vi "PolyGen.vi"() -> ()   [LabVIEW 2016]
uses:
  <vilib>/Utility/file.llb/Read Delimited Spreadsheet (string).vi
  <vilib>/Analysis/NI_AALPro.lvlib
panel:
  out "Z":cluster{dbl, dbl[]}[](array[cluster])
  out "X":cluster{dbl, dbl[]}[](array[cluster])
  out "Y":cluster{dbl, dbl[]}[](array[cluster])
  out "Application:Command Line Arguments":string[](array[string])
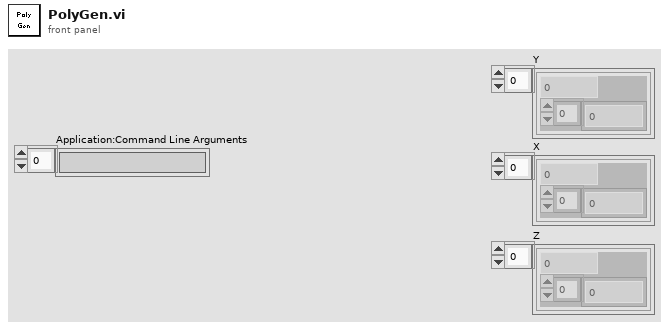
[diagram p1: front panel]
types:
  T1 = enum16{"open", "replace", "create", "open or create", "replace or create", "replace or create with confirmation"}
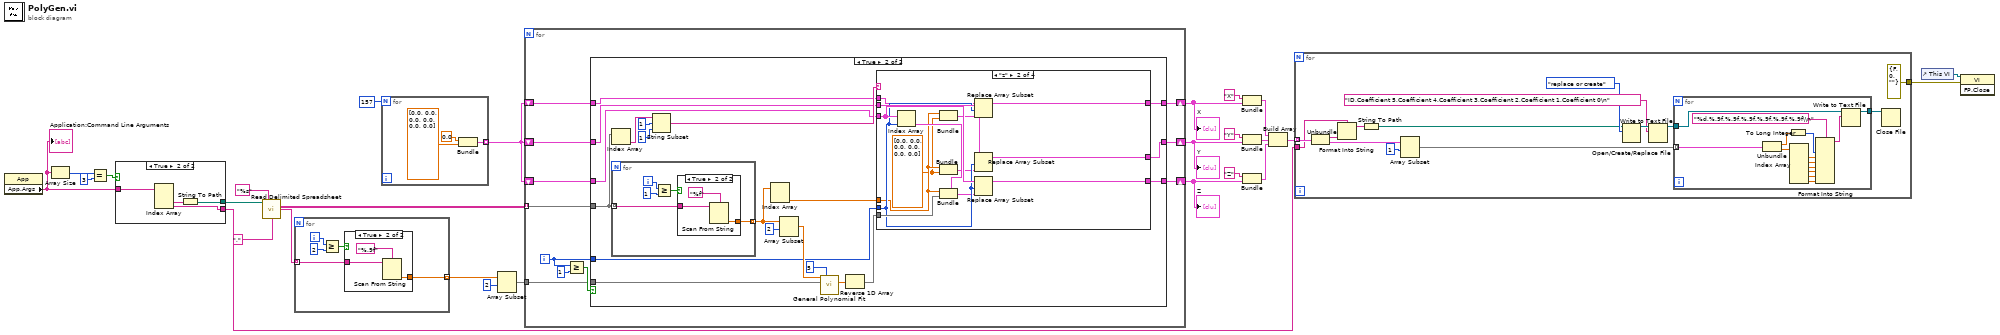
[diagram p0: block diagram]
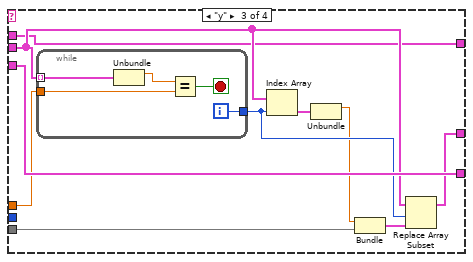
[diagram p4: hidden frame]
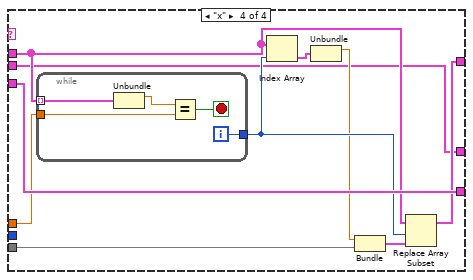
[diagram p5: hidden frame]
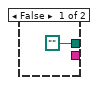
[diagram p8: hidden frame]
diagram:
  n1 = property class="App"() -> ("App.Args"=w24:string[])  [unwired: 2 in, 2 out]
  "Application:Command Line Arguments" <- w24
  n2 = Array Size(array=w24) -> (size(s)=w23:i32)
  n3 = Equal?(x=w23, y=3) -> (x = y?=w21:bool)
  n4 = case shown="True" w21 {
    tunnel: w24 -> [_ w32]
    tunnel: [path "" w31] -> w25
    tunnel: [_ w29] -> w3
    frame False {
    }
    frame True {
      n5 = Index Array(array=w32) -> (element #2=w30:string, element #3=w29:string)  [unwired: 3 in, 1 out]
      n6 = String To Path(string=w30) -> (path=w31:path)
    }
  }
  n7 = call-poly <vilib>:"Read Delimited Spreadsheet.vi"("file path (dialog if empty)"=w25, "format (%s)"="%s", "delimiter (\\t)"="," ("delimiter (\\t)")) -> ("all rows"=w17:string[][], "first row"=w20:string[])  [unwired: 7 in, 4 out]
  n8 = for {
    tunnel: w20 -> [w34] mode=indexing
    tunnel: [w33] -> w19 mode=indexing
    i -> [w37]
    n9 = Greater Or Equal?(x=w37, y=2) -> (x >= y?=w35:bool)
    n10 = case shown="True" w35 {
      tunnel: w34 -> [_ w40]
      tunnel: [_ w38] -> w33
      frame False {
      }
      frame True {
        n11 = Scan From String(format string="%.9f", input string=w40) -> (output 1=w38:dbl)  [unwired: 3 in, 3 out]
      }
    }
  }
  n12 = for {
    N: 157 -> [_]
    tunnel: [w41] -> w15 mode=indexing
    n13 = Bundle(0.0, dbl[] [0.0, 0.0, 0.0, 0.0, 0.0, 0.0]) -> (w41:cluster{dbl, dbl[]})  [unwired: 1 in]
  }
  n14 = Array Subset(array=w19, index=2) -> (w16:dbl[])  [unwired: 1 in]
  n15 = for {
    tunnel: w17 -> [w52] mode=indexing
    tunnel: w16 -> [w51]
    shift-right: [w49] -> w8
    shift-left: w15 -> [w50]
    shift-right: [w46] -> w9
    shift-left: w15 -> [w47]
    shift-right: [w45] -> w10
    shift-left: w15 -> [w44]
    i -> [w48]
    n16 = Greater Or Equal?(x=w48, y=1) -> (x >= y?=w53:bool)
    n17 = case shown="True" w53 {
      tunnel: w52 -> [_ w71]
      tunnel: w51 -> [_ w75]
      tunnel: w50 -> [w55 w66]
      tunnel: [w55 w65] -> w49
      tunnel: w48 -> [_ w64]
      tunnel: w47 -> [w57 w61]
      tunnel: [w57 w60] -> w46
      tunnel: [w56 w59] -> w45
      tunnel: w44 -> [w56 w58]
      frame False {
      }
      frame True {
        n18 = Index Array(array=w71) -> (element=w70:string)  [unwired: 1 in]
        n19 = for {
          tunnel: w71 -> [w127] mode=indexing
          tunnel: [w126] -> w74 mode=indexing
          i -> [w129]
          n20 = Greater Or Equal?(x=w129, y=1) -> (x >= y?=w128:bool)
          n21 = case shown="True" w128 {
            tunnel: w127 -> [_ w131]
            tunnel: [_ w130] -> w126
            frame False {
            }
            frame True {
              n22 = Scan From String(format string="%f", input string=w131) -> (output 1=w130:dbl)  [unwired: 3 in, 3 out]
            }
          }
        }
        n23 = String Subset(string=w70, offset (0)=1, length (rest)=1 ("length (rest)")) -> (substring=w67:string)
        n24 = Index Array(array=w74) -> (element #2=w63:dbl)  [unwired: 2 in, 1 out]
        n25 = Array Subset(array=w74, index=2) -> (w76:dbl[])  [unwired: 1 in]
        n26 = call <vilib>:"General Polynomial Fit.vi"("Y"=w76, "polynomial order"=5, "X"=w75) -> ("Polynomial Coefficients"=w72:dbl[])  [unwired: 9 in, 3 out]
        n27 = Reverse 1D Array(array=w72) -> (reversed array=w62:dbl[])
        n28 = case shown="\"z\"" w67 {
          tunnel: w66 -> [w80 w92 w104 w119]
          tunnel: [w80 w85 w104 w119] -> w65
          tunnel: w64 -> [_ w89 _ _]
          tunnel: w63 -> [_ w84 w103 w118]
          tunnel: w62 -> [_ w93 w99 w115]
          tunnel: w61 -> [w79 w91 w102 w110]
          tunnel: [w79 w90 w96 w110] -> w60
          tunnel: [w78 w87 w95 w112] -> w59
          tunnel: w58 -> [w78 w88 w95 w111]
          frame "False", Default {
          }
          frame "z" {
            w83 = dbl[] [0.0, 0.0, 0.0, 0.0, 0.0, 0.0]
            n29 = Index Array(array=w92, index=w89) -> (element=w94:cluster{dbl, dbl[]})
            n30 = Bundle(w84, w83) -> (w81:cluster{dbl, dbl[]})  [unwired: 1 in]
            n31 = Bundle(w84, w83) -> (w82:cluster{dbl, dbl[]})  [unwired: 1 in]
            n32 = Bundle(cluster=w94, w84, w93) -> (w86:cluster{dbl, dbl[]})
            n33 = Replace Array Subset(array=w88, new element=w81, index=w89) -> (w87:cluster{dbl, dbl[]}[])
            n34 = Replace Array Subset(array=w91, new element=w82, index=w89) -> (w90:cluster{dbl, dbl[]}[])
            n35 = Replace Array Subset(array=w92, new element=w86, index=w89) -> (w85:cluster{dbl, dbl[]}[])
          }
          frame "y" {
            n36 = while {
              tunnel: w103 -> [w106]
              tunnel: w102 -> [w109] mode=indexing
              tunnel: [w108] -> w101
              i -> [w108]
              stop <- w105 stop-if-true
              n37 = Unbundle(w109) -> (w107:dbl)  [unwired: 1 out]
              n38 = Equal?(x=w107, y=w106) -> (x = y?=w105:bool)
            }
            n39 = Index Array(array=w102, index=w101) -> (element=w100:cluster{dbl, dbl[]})
            n40 = Unbundle(w100) -> (w98:dbl)  [unwired: 1 out]
            n41 = Bundle(w98, w99) -> (w97:cluster{dbl, dbl[]})  [unwired: 1 in]
            n42 = Replace Array Subset(array=w102, new element=w97, index=w101) -> (w96:cluster{dbl, dbl[]}[])
          }
          frame "x" {
            n43 = while {
              tunnel: w118 -> [w121]
              tunnel: w111 -> [w124] mode=indexing
              tunnel: [w123] -> w117
              i -> [w123]
              stop <- w120 stop-if-true
              n44 = Unbundle(w124) -> (w122:dbl)  [unwired: 1 out]
              n45 = Equal?(x=w122, y=w121) -> (x = y?=w120:bool)
            }
            n46 = Index Array(array=w111, index=w117) -> (element=w116:cluster{dbl, dbl[]})
            n47 = Unbundle(w116) -> (w114:dbl)  [unwired: 1 out]
            n48 = Bundle(w114, w115) -> (w113:cluster{dbl, dbl[]})  [unwired: 1 in]
            n49 = Replace Array Subset(array=w111, new element=w113, index=w117) -> (w112:cluster{dbl, dbl[]}[])
          }
        }
      }
    }
  }
  "Y" <- w9
  "X" <- w10
  "Z" <- w8
  n50 = Bundle("X", w10) -> (w7:cluster{string, cluster{dbl, dbl[]}[]})  [unwired: 1 in]
  n51 = Bundle("Y", w9) -> (w6:cluster{string, cluster{dbl, dbl[]}[]})  [unwired: 1 in]
  n52 = Bundle("Z", w8) -> (w5:cluster{string, cluster{dbl, dbl[]}[]})  [unwired: 1 in]
  n53 = Build Array(w7, w6, w5) -> (w4:cluster{string, cluster{dbl, dbl[]}[]}[])
  n54 = for {
    tunnel: w4 -> [w146] mode=indexing
    tunnel: w3 -> [w145]
    tunnel: [errorcluster {"status"=FALSE, "code"=0, "source"=""} ("error in (no error)")] -> w1
    n55 = Unbundle(w146) -> (w144:string, w138:cluster{dbl, dbl[]}[])
    n56 = Format Into String(format string=w145, w144) -> (resulting string=w143:string)  [unwired: 2 in, 1 out]
    n57 = String To Path(string=w143) -> (path=w141:path)
    n58 = Array Subset(array=w138, index=1) -> (w136:cluster{dbl, dbl[]}[])  [unwired: 1 in]
    n59 = Open/Create/Replace File(file path (use dialog)=w141, operation (0:open)=T1."replace or create") -> (refnum out=w140:refnum<file>)  [unwired: 4 in, 2 out]
    n60 = Write to Text File(file (use dialog)=w140, text="ID,Coefficient 5,Coefficient 4,Coefficient 3,Coefficient 2,Coefficient 1,Coefficient 0\n") -> (refnum out=w135:refnum<file>)  [unwired: 2 in, 2 out]
    n61 = for {
      tunnel: w136 -> [w159] mode=indexing
      tunnel: w135 -> [w148]
      tunnel: [w147] -> w134
      n62 = Unbundle(w159) -> (w157:dbl, w158:dbl[])
      n63 = To Long Integer(number=w157) -> (32bit integer=w156:i32)
      n64 = Index Array(array=w158) -> (element #1=w155:dbl, element #2=w154:dbl, element #3=w153:dbl, element #4=w152:dbl, element #5=w151:dbl, element #6=w150:dbl)  [unwired: 6 in]
      n65 = Format Into String(format string="%d,%.9f,%.9f,%.9f,%.9f,%.9f,%.9f\\n", w156, w155, w154, w153, w152, w151, w150) -> (resulting string=w149:string)  [unwired: 2 in, 1 out]
      n66 = Write to Text File(file (use dialog)=w148, text=w149) -> (refnum out=w147:refnum<file>)  [unwired: 2 in, 2 out]
    }
    n67 = Close File(refnum=w134) -> ()  [unwired: 1 in, 2 out]
  }
  n68 = control-ref of="This VI"() -> (w2:refnum<vi>)
  n69 = invoke class="VI" method="FP.Close"(reference=w2, error in=w1) -> ()  [unwired: 1 in, 3 out]
